vi "Update Connection Cache.vi"(6 "Connection Reference":refnum<data-value>, 11 "ConnectionFactoryHandler in":refnum<class "ConnectionFactoryHandler.lvclass">) -> (3 "ConnectionFactoryHandler out":refnum<class "ConnectionFactoryHandler.lvclass">)   [LabVIEW 2020, in "ConnectionFactorySession.lvlib" / "ConnectionFactoryHandler.lvclass"]
uses:
  <vilib>/gpm_packages/@cs/Network-interface/Source/Connection Factory Session/ConnectionFactoryHandler/ConnectionFactoryHandler.lvclass
  <vilib>/gpm_packages/@cs/Network-interface/Source/Connection Reference/Connection Reference/Connection Reference.lvclass
  <vilib>/gpm_packages/@cs/Network-interface/Source/Connection Factory Session/ConnectionFactoryHandler/ConnectionFactoryHandler.lvclass/ConnectionFactoryHandler.ctl
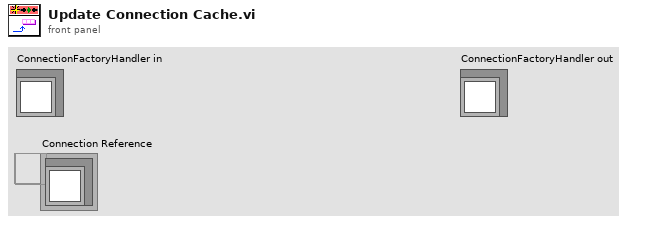
[diagram p1: front panel]
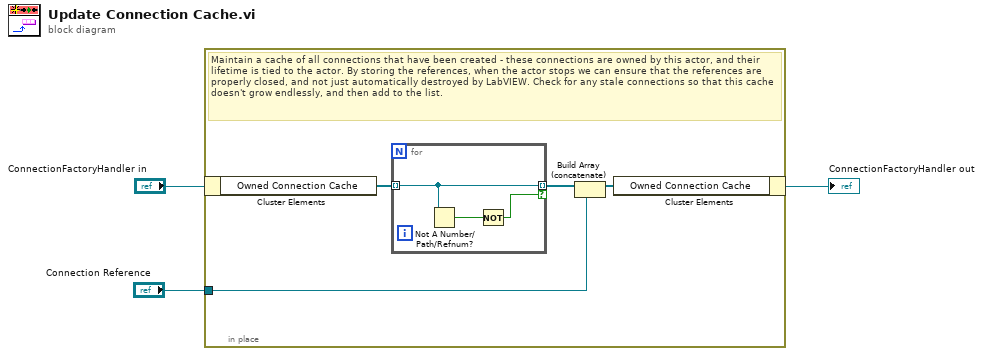
[diagram p0: block diagram]
diagram:
  n1 = in-place {
    in-place-border: "Connection Reference" -> [w4]
    # "Maintain a cache of all connections that have been created - these connections are owned by this actor, and their lifetime is tied to the actor. By storing the references, when the actor stops we can ensure that the references are properly closed, and not just automatically destroyed by LabVIEW. Check for any stale connections so that this cache doesn't grow endlessly, and then add to the list."
    n2 = in-place-cluster #1("ConnectionFactoryHandler in") -> ("Owned Connection Cache"=w7:refnum<data-value>[])
    n3 = for {
      tunnel: w7 -> [w10] mode=indexing
      tunnel: [w10] -> w6 mode=indexing if=w8
      n4 = Not A Number/Path/Refnum?(number/path/refnum=w10) -> (NaN/Path/Refnum?=w9:bool)
      n5 = Not(x=w9) -> (.not. x?=w8:bool)
    }
    n6 = Build Array (concatenate)(w6, w4) -> (w5:refnum<data-value>[])
    n7 = in-place-cluster #1("Owned Connection Cache"=w5) -> (→"ConnectionFactoryHandler out":refnum<class "ConnectionFactoryHandler.lvclass">)
  }
